vi "SetSize.vi"(0 "时频域1":refnum<vi>, 1 "Choose1":refnum<vi>, 2 "录波开始时间":refnum<vi>, 3 "已录波":refnum<vi>, 5 "Graph1":refnum<vi>, 6 "XYGraph":refnum<vi>, 7 "FcdVI Refnum":refnum<vi>, 8 "Mode":refnum<vi>, 9 "Graph2":refnum<vi>, 11 "时频域2":refnum<vi>, 12 "Choose2":refnum<vi>, 13 "录波文件大小":refnum<vi>, 14 "录波？":refnum<vi>) -> ()   [LabVIEW 2014, in "Xgraph.xctl"]
uses:
  Xgraph.xctl
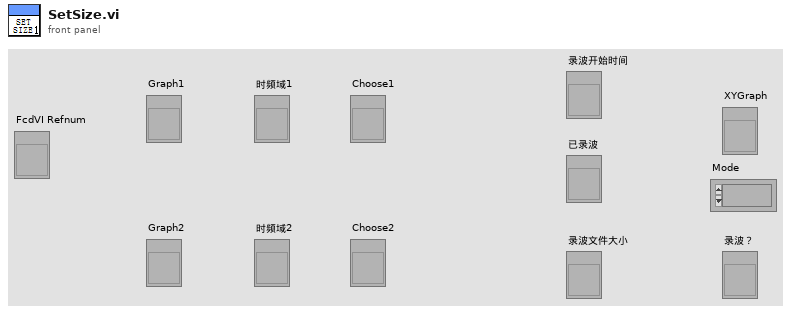
[diagram p1: front panel]
types:
  T1 = typedef "LVRectTypeDef.ctl" = cluster{"Left":i16, "Top":i16, "Right":i16, "Bottom":i16}
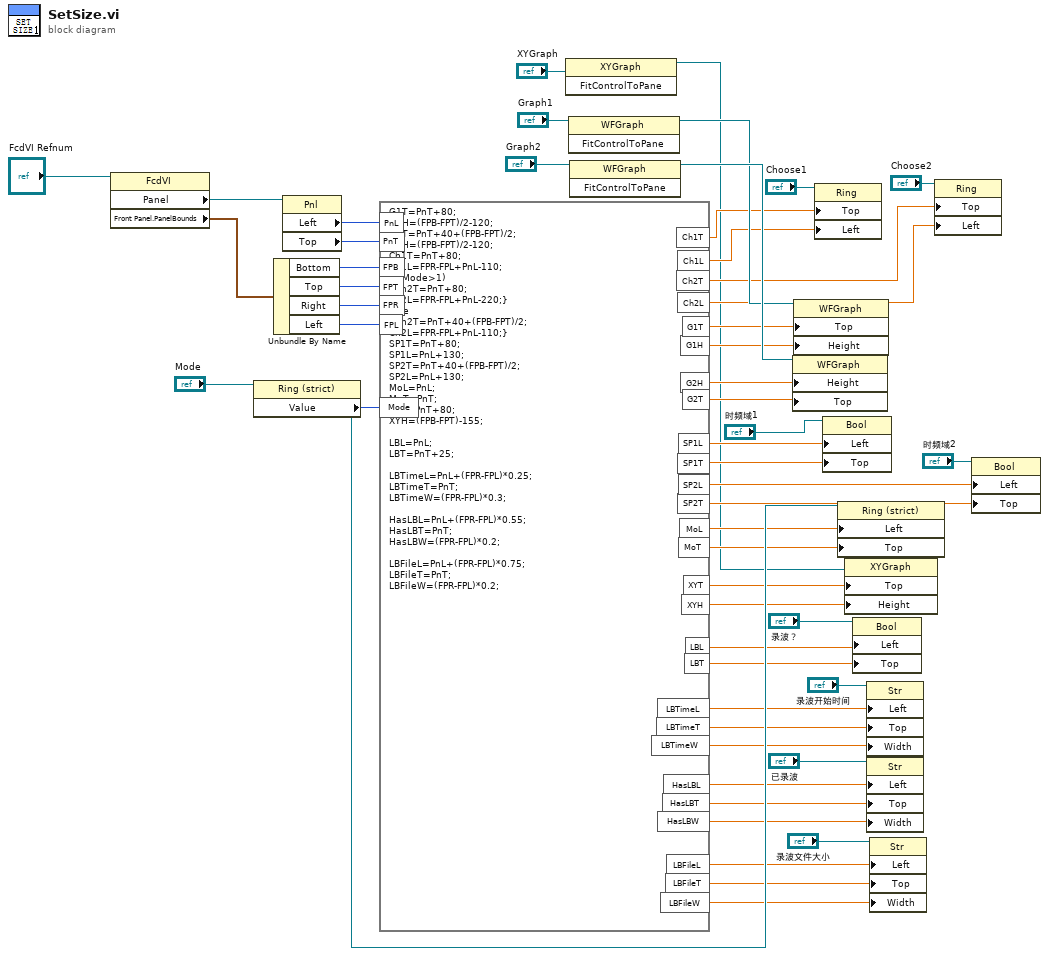
[diagram p0: block diagram]
diagram:
  n1 = property class="FcdVI"(reference="FcdVI Refnum") -> ("Panel"=w52:refnum<vi>, "Front Panel.PanelBounds"=w45:T1)  [unwired: 1 in, 2 out]
  n2 = property class="Ring (strict)"(reference="Mode") -> (reference out=w22:refnum<vi>, "Value"=w23:u16)  [unwired: 1 in, 1 out]
  n3 = Unbundle By Name(w45) -> ("Bottom"=w44:i16, "Top"=w43:i16, "Right"=w42:i16, "Left"=w41:i16)
  n4 = property class="Pnl"(reference=w52) -> ("Left"=w31:i32, "Top"=w40:i32)  [unwired: 1 in, 2 out]
  n5 = formula code="G1T=PnT+80;\nG1H=(FPB-FPT)/2-120;\nG2T=PnT+40+(FPB-FPT)/2;\nG2H=(FPB-FPT)/2-120;\nCh1T=PnT+80;\nCh1L=FPR-FPL+PnL-110;\nif (Mode>1)\n{Ch2T=PnT+80;\nCh2L=FPR-FPL+PnL-220;}\nelse\n{Ch2T=PnT+40+(FPB-FPT)/2;\nCh2L=FPR-FPL+PnL-110;}\nSP1T=PnT+80;\nSP1L=PnL+130;\nSP2T=PnT+40+(FPB-FPT)/2;\nSP2L=PnL+130;\nMoL=PnL;\nMoT=PnT;\nXYT=PnT+80;\nXYH=(FPB-FPT)-155;\n\nLBL=PnL;\nLBT=PnT+25;\n\nLBTimeL=PnL+(FPR-FPL)*0.25;\nLBTimeT=PnT;\nLBTimeW=(FPR-FPL)*0.3;\n\nHasLBL=PnL+(FPR-FPL)*0.55;\nHasLBT=PnT;\nHasLBW=(FPR-FPL)*0.2;\n\nLBFileL=PnL+(FPR-FPL)*0.75;\nLBFileT=PnT;\nLBFileW=(FPR-FPL)*0.2;"("FPB"=w44, "FPT"=w43, "FPR"=w42, "FPL"=w41, "PnT"=w40, "PnL"=w31, "Mode"=w23) -> ("G1H"=w37:dbl, "G2H"=w38:dbl, "G1T"=w36:dbl, "G2T"=w39:dbl, "Ch1T"=w35:dbl, "Ch1L"=w34:dbl, "Ch2T"=w33:dbl, "Ch2L"=w32:dbl, "SP1T"=w27:dbl, "SP1L"=w28:dbl, "SP2T"=w26:dbl, "SP2L"=w25:dbl, "MoL"=w21:dbl, "MoT"=w20:dbl, "XYT"=w19:dbl, "XYH"=w18:dbl, "LBL"=w14:dbl, "LBT"=w13:dbl, "LBTimeL"=w11:dbl, "LBTimeT"=w10:dbl, "LBFileL"=w5:dbl, "LBFileT"=w4:dbl, "HasLBL"=w8:dbl, "HasLBT"=w7:dbl, "LBTimeW"=w3:dbl, "HasLBW"=w2:dbl, "LBFileW"=w1:dbl)
  n6 = invoke class="XYGraph" method="FitControlToPane"(reference="XYGraph") -> (reference out=w16:refnum<vi>)  [unwired: 2 in, 2 out]
  n7 = invoke class="WFGraph" method="FitControlToPane"(reference="Graph1") -> (reference out=w50:refnum<vi>)  [unwired: 2 in, 2 out]
  n8 = invoke class="WFGraph" method="FitControlToPane"(reference="Graph2") -> (reference out=w51:refnum<vi>)  [unwired: 2 in, 2 out]
  n9 = property class="WFGraph"(reference=w51, "Height"=w38, "Top"=w39) -> ()  [unwired: 1 in, 2 out]
  n10 = property class="WFGraph"(reference=w50, "Top"=w36, "Height"=w37) -> ()  [unwired: 1 in, 2 out]
  n11 = property class="Ring"(reference="Choose1", "Top"=w35, "Left"=w34) -> ()  [unwired: 1 in, 2 out]
  n12 = property class="Bool"(reference="时频域1", "Left"=w28, "Top"=w27) -> ()  [unwired: 1 in, 2 out]
  n13 = property class="Ring (strict)"(reference=w22, "Left"=w21, "Top"=w20) -> ()  [unwired: 1 in, 2 out]
  n14 = property class="XYGraph"(reference=w16, "Top"=w19, "Height"=w18) -> ()  [unwired: 1 in, 2 out]
  n15 = property class="Bool"(reference="录波？", "Left"=w14, "Top"=w13) -> ()  [unwired: 1 in, 2 out]
  n16 = property class="Str"(reference="录波开始时间", "Left"=w11, "Top"=w10, "Width"=w3) -> ()  [unwired: 1 in, 2 out]
  n17 = property class="Str"(reference="已录波", "Left"=w8, "Top"=w7, "Width"=w2) -> ()  [unwired: 1 in, 2 out]
  n18 = property class="Str"(reference="录波文件大小", "Left"=w5, "Top"=w4, "Width"=w1) -> ()  [unwired: 1 in, 2 out]
  n19 = property class="Ring"(reference="Choose2", "Top"=w33, "Left"=w32) -> ()  [unwired: 1 in, 2 out]
  n20 = property class="Bool"(reference="时频域2", "Left"=w25, "Top"=w26) -> ()  [unwired: 1 in, 2 out]
